vi "Engine Start Val Change.vi"(8 "error in (no error)":errorcluster, 11 "Engine Start":T2 scale=0.0..2.0) -> (0 "error out":errorcluster)   [LabVIEW 2018]
doc: "This subVI enqueues the named action in to the communications queue along with the input data."
uses:
  Private Controls/Module Action.ctl
  Controller (Host).lvlib
  Private Controls/Module Data.ctl
  Testing UI 1/Public Controls/Engine Start Control.ctl
  Testing UI 1/Testing UI 1.lvlib
panel:
  in  "Action":T1=enum."Engine Start Val Change"
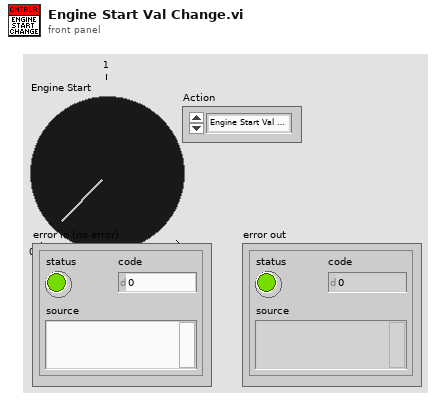
[diagram p1: front panel]
types:
  T1 = typedef "Controller (Host).lvlib/Module Action.ctl" = enum8{"Timeout", "Init", "Error", "Exit", "Set cRIO Connected Status", "Prompt Login", "Prompt Main Menu", "Prompt APU Select", "Prompt Operation Select", "Prompt SubTests Select", "Prompt Break Out", "Calibration", "Testing", "Load User Info", "Set Instr Init Status", "Load APU Setup Data", "Engine Start Val Change", "RPM Cross 95Perc Thresh", "Interactive Ctrls Val Change", "Update Report FilePath"}
  T2 = typedef "Testing UI 1.lvlib/Engine Start Control.ctl" = u8
  T3 = typedef "Controller (Host).lvlib/Module Data.ctl" = cluster{"Data":variant, "Action":T4}
  T4 = typedef "Controller (Host).lvlib/Module Action.ctl" = enum8{"Timeout", "Init", "Error", "Exit", "Set cRIO Connected Status", "Prompt Login", "Prompt Main Menu", "Prompt APU Select", "Prompt Operation Select", "Prompt SubTests Select", "Calibration", "Testing", "Load User Info", "Set Instr Init Status", "Load APU Setup Data", "RPM Cross 95Perc Thresh", "Interactive Ctrls Val Change", "Update Report FilePath"}
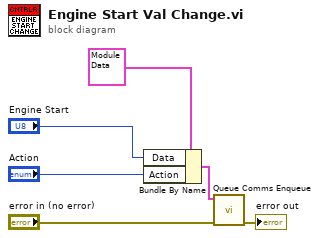
[diagram p0: block diagram]
diagram:
  n1 = Bundle By Name(cluster=T3 {"Data"=variant, "Action"=enum."Init"} ("element"), "Data"="Engine Start", "Action"="Action") -> (w5:T3)
  n2 = call "Queue Comms Enqueue.vi"("error in (no error)"="error in (no error)", "element"=w5) -> ("error out"=→"error out":errorcluster)  [unwired: 9 in]
